vi "Control General.vi"(10 "Baud Rate":u32=9600, 11 "VISA resource name":refnum<visa-resource-name>="COM13") -> ()   [LabVIEW 2013, in "Proyecto 2 Touch.lvrbt"]
uses:
  Proyecto 2 Touch.lvrbt
  <vilib>/Instr/_visa.llb/VISA Configure Serial Port (Instr).vi
  Global Var.vi
panel:
  out "Mensaje Completo":string
  out "X":i32
  out "Y":i32
  out "Z":i32
  out "Mensaje":string
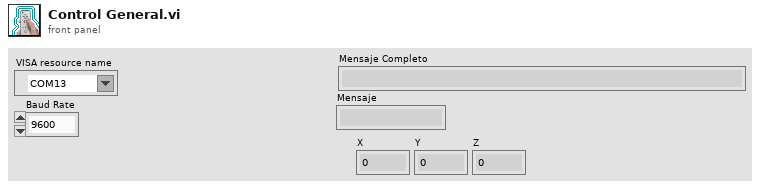
[diagram p1: front panel]
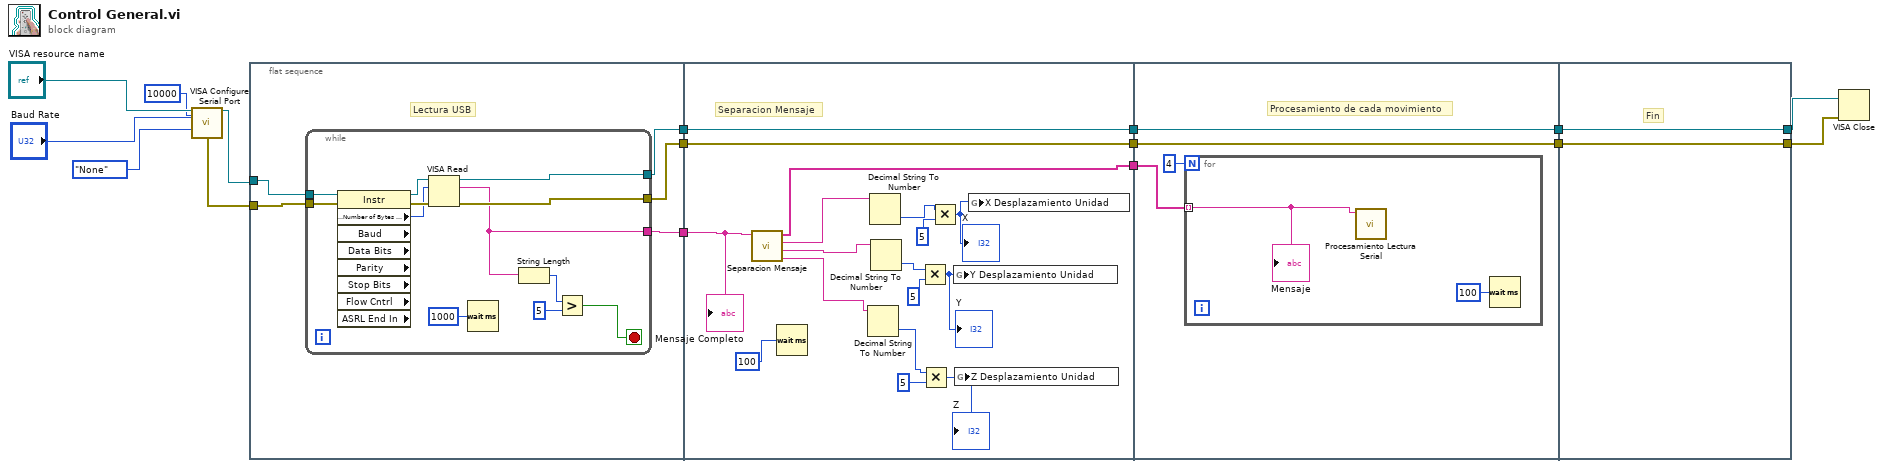
[diagram p0: block diagram]
diagram:
  n1 = call-poly "VISA Configure Serial Port"("VISA resource name"="VISA resource name", "timeout (10sec)"=u32 10000, "baud rate (9600)"="Baud Rate", "parity (0:none)"=enum16{"None", "Odd", "Even", "Mark", "Space"}."None") -> ("VISA resource name out"=w13:refnum<visa-resource-name>, "error out"=w12:errorcluster)  [unwired: 10 in]
  n2 = flat-sequence {
    tunnel: w13 -> [w21]
    tunnel: w12 -> [w20]
    tunnel: [w19] -> w8
    tunnel: [w18] -> w7
    tunnel: [w17] -> w6
    tunnel: w8 -> [w50]
    tunnel: w7 -> [w49]
    tunnel: w6 -> [w47]
    tunnel: [w50] -> w5
    tunnel: [w49] -> w4
    tunnel: [w43] -> w3
    tunnel: w5 -> [w54]
    tunnel: w4 -> [w53]
    tunnel: w3 -> [w51]
    tunnel: [w54] -> w2
    tunnel: [w53] -> w1
    tunnel: [w57] -> w10
    tunnel: [w58] -> w11
    tunnel: w2 -> [w58]
    tunnel: w1 -> [w57]
    frame #0 {
      # "Lectura USB"
      n3 = while {
        tunnel: w21 -> [w33]
        tunnel: w20 -> [w32]
        tunnel: [w31] -> w19
        tunnel: [w30] -> w18
        tunnel: [w22] -> w17
        stop <- w24 stop-if-true
        n4 = property class="Instr" props=["Serial Settings:Number of Bytes at Serial Port", "Baud", "Data Bits", "Parity", "Stop Bits", "Flow Cntrl", "ASRL End In"](reference=w33, error in=w32) -> (reference out=w29:refnum<visa-resource-name>, error out=w28:errorcluster, "Serial Settings:Number of Bytes at Serial Port"=w27:u32)  [unwired: 6 out]
        n5 = VISA Read(VISA resource name=w29, byte count=w27, error in (no error)=w28) -> (VISA resource name out=w31:refnum<visa-resource-name>, read buffer=w22:string, error out=w30:errorcluster)  [unwired: 1 out]
        n6 = Wait (ms)(milliseconds to wait=u32 1000) -> ()  [unwired: 1 out]
        n7 = String Length(string=w22) -> (length=w25:i32)
        n8 = Greater?(x=w25, y=5) -> (0:w24:bool)
      }
    }
    frame #1 {
      # "Separacion Mensaje"
      n9 = call "Separacion Mensaje.vi"("Mensaje"=w47) -> ("Z"=w44:string, "Y"=w45:string, "X"=w46:string, "Arreglo Entradas"=w43:string[])  [unwired: 7 in]
      n10 = Wait (ms)(milliseconds to wait=u32 100) -> ()  [unwired: 1 out]
      n11 = Decimal String To Number(string=w44) -> (number=w41:i32)  [unwired: 2 in, 1 out]
      n12 = Decimal String To Number(string=w46) -> (number=w35:i32)  [unwired: 2 in, 1 out]
      n13 = Decimal String To Number(string=w45) -> (number=w38:i32)  [unwired: 2 in, 1 out]
      n14 = Multiply(x=w38, y=5) -> (x*y=w39:i32)
      "Y" <- w39
      n15 = Multiply(x=w41, y=5) -> (x*y=w42:i32)
      "Z" <- w42
      n16 = Multiply(x=w35, y=5) -> (x*y=w34:i32)
      "X" <- w34
      n17 = global write "Global Var.vi" "Y Desplazamiento Unidad"(w39) -> ()
      n18 = global write "Global Var.vi" "Z Desplazamiento Unidad"(w42) -> ()
      n19 = global write "Global Var.vi" "X Desplazamiento Unidad"(w34) -> ()
      "Mensaje Completo" <- w47
    }
    frame #2 {
      # "Procesamiento de cada movimiento"
      n20 = for {
        N: 4 -> [_]
        tunnel: w51 -> [w55] mode=indexing
        n21 = call "Procesamiento Lectura Serial.vi"("Accion"=w55) -> ()  [unwired: 11 in]
        n22 = Wait (ms)(milliseconds to wait=u32 100) -> ()  [unwired: 1 out]
        "Mensaje" <- w55
      }
    }
    frame #3 {
      # "Fin"
    }
  }
  n23 = VISA Close(VISA resource name=w11, error in (no error)=w10) -> ()  [unwired: 1 out]
